vi "Initialize Parallel Events.vi"(8 "error in (no error)":errorcluster, 11 "CIFPluginManager in":refnum<class "CIFPluginManager.lvclass">) -> (0 "error out":errorcluster, 3 "CIFPluginManager out":refnum<class "CIFPluginManager.lvclass">)   [LabVIEW 2021, in "CIFPluginManager.lvclass"]
uses:
  CIFPluginManager.lvclass
  CIFPluginManager.lvclass/CIFPluginManager.ctl
  typedef/Loader Type.ctl
  typedef/Loader Load Info.ctl
  typedef/Plugin Load Info.ctl
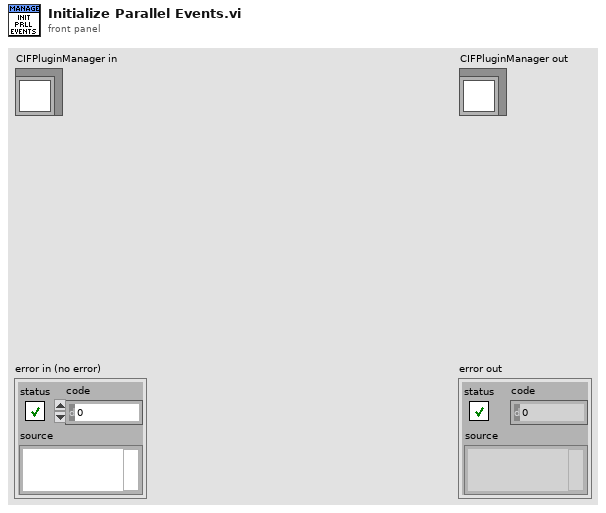
[diagram p1: front panel]
types:
  T1 = typedef "CIFPluginManager.lvclass/Plugin Load Info.ctl" = cluster{"Plugin Name":string, "Plugin Path":string, "Launcher Name":string, "Launcher Type":T2}
  T2 = typedef "CIFPluginManager.lvclass/Loader Type.ctl" = enum16{"LabVIEW"}
  T3 = typedef "CIFPluginManager.lvclass/Loader Load Info.ctl" = cluster{"Loader Type":T2, "Loader Name":string}
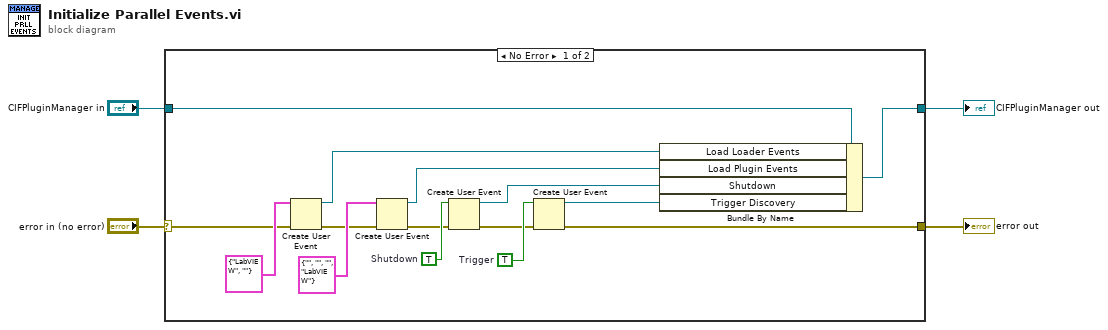
[diagram p0: block diagram]
diagram:
  n1 = case shown="No Error" "error in (no error)" {
    selector: "error in (no error)" -> [w5 w21]
    tunnel: [w12 w21] -> w3
    tunnel: [w18 w20] -> w1
    tunnel: "CIFPluginManager in" -> [w19 w20]
    frame No Error {
      w14 = TRUE  # Shutdown
      w17 = TRUE  # Trigger
      n2 = Create User Event(user event datatype=T3 {"Loader Type"=enum."LabVIEW", "Loader Name"=""} ("Launcher Load Info"), error in=w5) -> (user event=w10:refnum<user-event>, error out=w6:errorcluster)
      n3 = Create User Event(user event datatype=T1 {"Plugin Name"="", "Plugin Path"="", "Launcher Name"="", "Launcher Type"=enum."LabVIEW"} ("Plugin Load Info"), error in=w6) -> (user event=w8:refnum<user-event>, error out=w7:errorcluster)
      n4 = Create User Event(user event datatype=w14, error in=w7) -> (user event=w13:refnum<user-event>, error out=w15:errorcluster)
      n5 = Create User Event(user event datatype=w17, error in=w15) -> (user event=w16:refnum<user-event>, error out=w12:errorcluster)
      n6 = Bundle By Name(cluster=w19, "Load Loader Events"=w10, "Load Plugin Events"=w8, "Shutdown"=w13, "Trigger Discovery"=w16) -> (w18:refnum<class "CIFPluginManager.lvclass">)
    }
    frame Error {
    }
  }
  "error out" <- w3
  "CIFPluginManager out" <- w1
